vi "Convert UI Connection to Connection (R,S,D).vi.vi"(11 "Connection":T1) -> (3 "Connection (R,S,D)":T2)   [LabVIEW 2017, in "Routing and Faulting System Explorer.lvlib"]
uses:
  Routing and Faulting System Explorer.lvlib
  Shared/Connection.ctl
  Connection Row.ctl
  Shared/Routing and Faulting Shared.lvlib
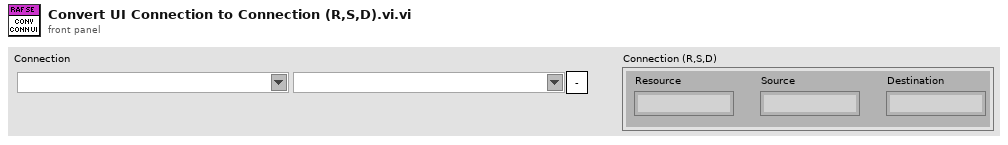
[diagram p1: front panel]
types:
  T1 = typedef "Routing and Faulting System Explorer.lvlib/Connection Row.ctl" = cluster{"Source":string, "Destination":string, "Remove":bool}
  T2 = typedef "Routing and Faulting Shared.lvlib/Connection.ctl" = cluster{"Resource":string, "Source":string, "Destination":string}
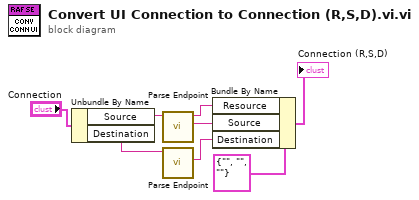
[diagram p0: block diagram]
diagram:
  n1 = Unbundle By Name("Connection") -> ("Source"=w2:string, "Destination"=w6:string)
  n2 = call "Parse Endpoint.vi"("Resource/Endpoint"=w2) -> ("Endpoint"=w5:string, "Resource"=w4:string)  [unwired: 9 in]
  n3 = call "Parse Endpoint.vi"("Resource/Endpoint"=w6) -> ("Endpoint"=w7:string)  [unwired: 9 in, 1 out]
  n4 = Bundle By Name(cluster=T2 {"Resource"="", "Source"="", "Destination"=""} ("Connection (R,S,D)"), "Resource"=w4, "Source"=w5, "Destination"=w7) -> (→"Connection (R,S,D)":T2)
